vi "Caraya simple approval test.vi"   [LabVIEW 2020]
uses:
  <vilib>/SAS/Approval Tests/Pass If Approved.vi
  MyTestCase/MyTestCase.lvclass
  <vilib>/addons/_JKI Toolkits/Caraya/classes/Test/Test.lvclass
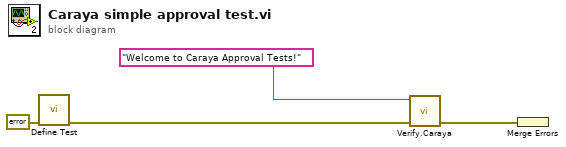
[diagram p0: block diagram]
diagram:
  n1 = call <vilib>:"Define Test.vi"("error in (no error)"=errorcluster {"status"=FALSE, "code"=0, "source"=""}) -> ("error out"=w2:errorcluster)  [unwired: 9 in, 1 out]
  n2 = call "Verify.Caraya.vi"("error in (no error)"=w2, "Test Data"="Welcome to Caraya Approval Tests!") -> ("error out"=w1:errorcluster)  [unwired: 9 in]
  n3 = Merge Errors(w1) -> ()  [unwired: 1 out]
